vi "teste_math_return.vi"() -> ()   [LabVIEW 2019]
uses:
  <instrlib>/Yokogawa PZ4000/Yokogawa PZ4000.lvlib
panel:
  out "substring":string
  out "*(type *) &x":i16[](array[numeric])
  out "Data Byte Number":i32
  out "Precision":i16
  out "read buffer":string
  out "Waveform Graph":u32[](graph)
  in  "error in (no error)":errorcluster
  in  "VISA resource name":refnum<visa-resource-name>
  in  "Start Point (0)":u32 max=4000000 step=1
  in  "End Point (1000)":u32=1000 max=4000000 step=1
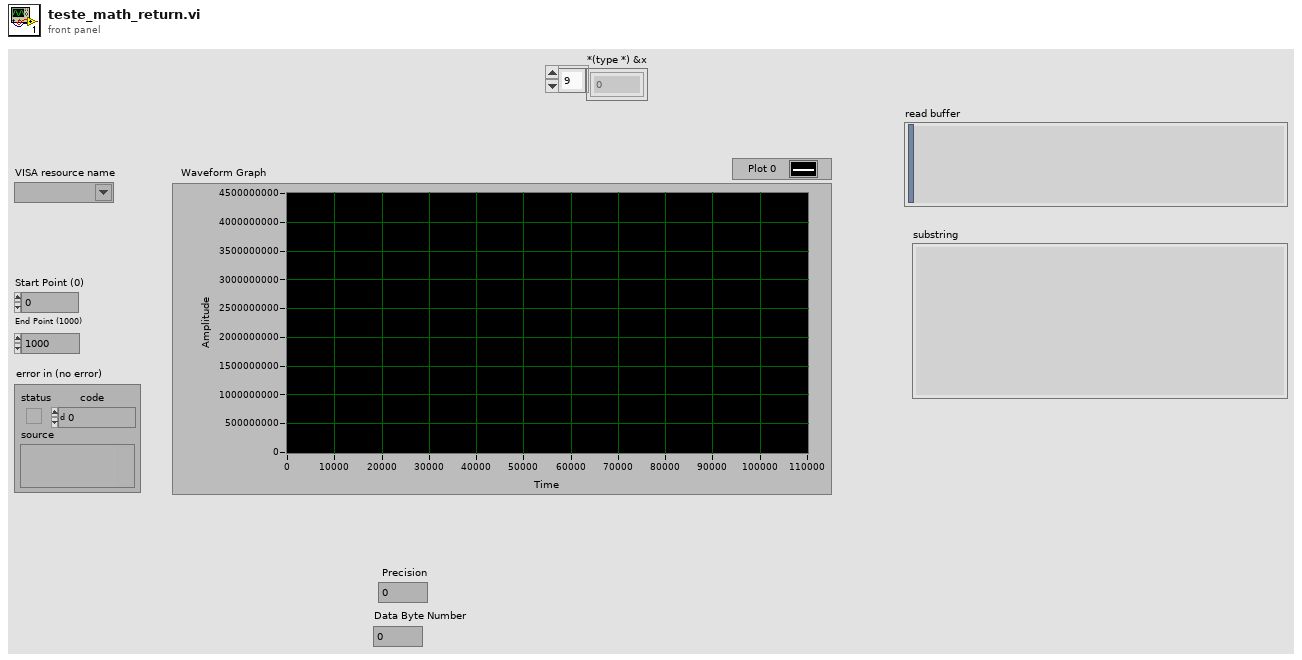
[diagram p1: front panel]
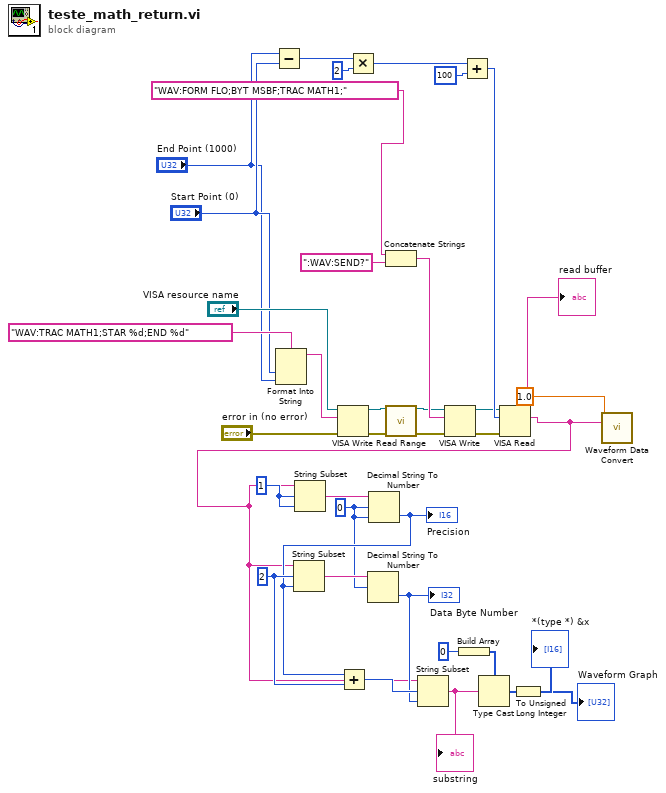
[diagram p0: block diagram]
diagram:
  w14 = 2
  w8 = 1
  w3 = i16 0
  n1 = Subtract(x="End Point (1000)", y="Start Point (0)") -> (x-y=w29:u32)
  n2 = Format Into String(format string="WAV:TRAC MATH1;STAR %d;END %d", "Start Point (0)", "End Point (1000)") -> (resulting string=w32:string)  [unwired: 2 in, 1 out]
  n3 = VISA Write(VISA resource name="VISA resource name", write buffer=w32, error in (no error)="error in (no error)") -> (VISA resource name out=w31:refnum<visa-resource-name>, error out=w30:errorcluster)  [unwired: 1 out]
  n4 = Multiply(x=w29, y=u32 2) -> (x*y=w27:u32)
  n5 = Concatenate Strings("WAV:FORM FLO;BYT MSBF;TRAC MATH1;", ":WAV:SEND?") -> (w22:string)
  n6 = call <instrlib>:"Read Range.vi"("VISA resource name"=w31, "error in (no error)"=w30) -> ("VISA resource name out"=w20:refnum<visa-resource-name>, "error out"=w19:errorcluster)  [unwired: 11 in, 1 out]
  n7 = VISA Write(VISA resource name=w20, write buffer=w22, error in (no error)=w19) -> (VISA resource name out=w23:refnum<visa-resource-name>, error out=w25:errorcluster)  [unwired: 1 out]
  n8 = Build Array(i16 0) -> (w6:i16[])
  n9 = Add(x=w27, y=u32 100) -> (x+y=w24:u32)
  n10 = VISA Read(VISA resource name=w23, byte count=w24, error in (no error)=w25) -> (read buffer=w2:string)  [unwired: 3 out]
  "read buffer" <- w2
  n11 = String Subset(string=w2, offset (0)=w8, length (rest)=w8) -> (substring=w12:string)
  n12 = Decimal String To Number(string=w12, offset=w3, default (0L)=w3) -> (number=w10:i16)  [unwired: 1 out]
  "Precision" <- w10
  n13 = String Subset(string=w2, offset (0)=w14, length (rest)=w10) -> (substring=w13:string)
  n14 = Add(x=w10, y=w14) -> (x+y=w11:i32)
  n15 = Decimal String To Number(string=w13, offset=w3) -> (number=w9:i32)  [unwired: 1 in, 1 out]
  "Data Byte Number" <- w9
  n16 = String Subset(string=w2, offset (0)=w11, length (rest)=w9) -> (substring=w4:string)
  "substring" <- w4
  n17 = Type Cast(type=w6, x=w4) -> (*(type *) &x=w5:i16[])
  "*(type *) &x" <- w5
  n18 = To Unsigned Long Integer(number=w5) -> (unsigned 32bit integer=→"Waveform Graph":u32[])
  n19 = call <instrlib>:"Waveform Data Convert.vi"("Input Data"=w2, "Range"=1.0) -> ()  [unwired: 11 in, 3 out]
